vi "Teleop.vi"(10 "Match Info":T1={"Autonomous Elapsed Seconds"=0.0, "TeleOp Elapsed Seconds"=0.0, "Disabled Elapsed Seconds"=0.0, "Visited Autonomous"=FALSE, "Visited TeleOp"=FALSE, "Visited Disabled"=FALSE, "Autonomous Settings"={"Autonomous Style"=enum."Independent", "VI Refnum"=refnum}}, 11 "Call Context":T2) -> ()   [LabVIEW 2015]
doc: "This VI is called for each TeleOp packet received from the DS where the robot is not disabled. It is often used to read from the joysticks and update I/O or to update setpoints for timed control loops. It should complete and return within 20 milliseconds or it may miss DS packets."
uses:
  Robot Global Data.vi
  AppleScript/AppleScript Global Data.vi
  <vilib>/Rock Robotics/Network Tables/NT Read Number.vi
  <vilib>/Rock Robotics/WPI/DriverStation/WPI_DriverStationMatch Info.ctl
  <vilib>/Rock Robotics/WPI/DriverStation/WPI_DriverStationDerivedRobotMode.ctl
panel:
  out "Distance":dbl
  in  "reset":bool
  out "Yaw":dbl
  in  "milliseconds to wait":u32=10
  out "x-y":u32
  in  "inactive":dbl=1.0
  in  "active":dbl
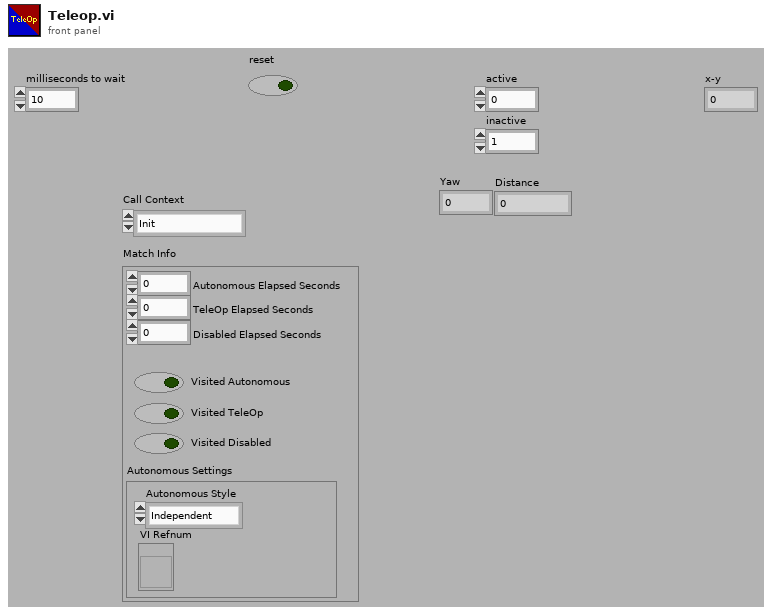
[diagram p1: front panel]
types:
  T1 = typedef "WPI_DriverStationMatch Info.ctl" = cluster{"Autonomous Elapsed Seconds":dbl, "TeleOp Elapsed Seconds":dbl, "Disabled Elapsed Seconds":dbl, "Visited Autonomous":bool, "Visited TeleOp":bool, "Visited Disabled":bool, "Autonomous Settings":cluster{"Autonomous Style":enum16{"Iterative", "Independent"}, "VI Refnum":refnum<vi>}}
  T2 = typedef "WPI_DriverStationDerivedRobotMode.ctl" = enum16{"Init", "Execute", "Stop"}
  T3 = typedef "WPI_JoystickDevRef.ctl" = cluster{"Device":T4}
  T4 = typedef "WPI_JoystickDeviceEnum.ctl" = enum16{"USB 0", "USB 1", "USB 2", "USB 3", "USB 4", "USB 5"}
  T5 = typedef "WPI_RobotDriveDevRef.ctl" = cluster{"DevStatus":errorcluster, "Motors[]":T6[], "Square Inputs":bool, "Max Output":dbl}
  T6 = typedef "WPI_MotorControlDeviceRef.ctl" = cluster{"DeviceStatus":errorcluster, "Type":T7, "PWM":cluster{"PWM Channel":T8, "DeadBand":T9}, "CAN":cluster{"Device Number":u8, "Control Mode":T10, "Semaphore":T11, "Max Vout":dbl, "TalonSRX Control Mode":T12}, "Invert":bool}
  T7 = typedef "WPI_MotorControlType.ctl" = enum16{"PWM", "CAN", "CANTalonSRX"}
  T8 = typedef "FPGA_DIOPWMChannel.ctl" = enum8{"PWM 0", "PWM 1", "PWM 2", "PWM 3", "PWM 4", "PWM 5", "PWM 6", "PWM 7", "PWM 8", "PWM 9", "PWM MXP 0", "PWM MXP 1", "PWM MXP 2", "PWM MXP 3", "PWM MXP 4", "PWM MXP 5", "PWM MXP 6", "PWM MXP 7", "PWM MXP 8", "PWM MXP 9", "Invalid"}
  T9 = typedef "WPI_PWMDeadband.ctl" = cluster{"Name":string, "maxPositivePwm":i32, "minPositivePwm":i32, "centerPwm":i32, "maxNegativePwm":i32, "minNegativePwm":i32, "angularRange":u16}
  T10 = typedef "WPI_CANJaguar_ControlMode.ctl" = enum8{"Percent VBus", "Current", "Speed", "Position", "Voltage"}
  T11 = typedef "Semaphore RefNum" = refnum<k1>
  T12 = typedef "WPI_CANTalonSRX_APIControlMode.ctl" = enum8{"Percent VBus", "Speed", "Position", "Slave", "Unchanged / Invalid", "Voltage Compensation", "Current", "Motion Profile"}
  T13 = typedef "WPI_ServoDeviceRef.ctl" = cluster{"DeviceStatus":errorcluster, "PWM Channel":T8, "DeadBand":T9}
  T14 = typedef "navX Library v2.lvlib/Z900_navX_DeviceTypeDef.ctl" = cluster{"Interface":cluster{"Protocol":T15, "Update Rate (4Hz-60Hz)":u8, "navX Open TypeDef":variant}, "Notify Packet":refnum<notifier>, "Loop VI Refnum":refnum<vi>, "Ready to Close Occurrence Refnum":refnum<k4>}
  T15 = typedef "navX Library v2.lvlib/Z900_navX_ProtocolTypeDef.ctl" = enum16{"SERIAL", "I2C", "SPI"}
  T16 = typedef "WPI_EncoderDevRef.ctl" = cluster{"DevStatus":errorcluster, "EncoderIndex":T17, "CounterIndex":T18, "DistancePerCount":dbl, "Decoding Type":T19}
  T17 = typedef "FPGA_EncoderIdx.ctl" = enum8{"Enc 0", "Enc 1", "Enc 2", "Enc 3", "Enc 4", "Enc 5", "Enc 6", "Enc 7", "Invalid"}
  T18 = typedef "FPGA_CounterCtrSystemIndex.ctl" = enum8{"Ctr 0", "Ctr 1", "Ctr 2", "Ctr 3", "Ctr 4", "Ctr 5", "Ctr 6", "Ctr 7", "Invalid"}
  T19 = typedef "WPI_EncoderType.ctl" = enum16{"1x", "2x", "4x"}
  T20 = cluster{"Yaw":dbl, "Roll":dbl, "Pitch":dbl, "Heading":dbl, "Fused Heading":dbl}
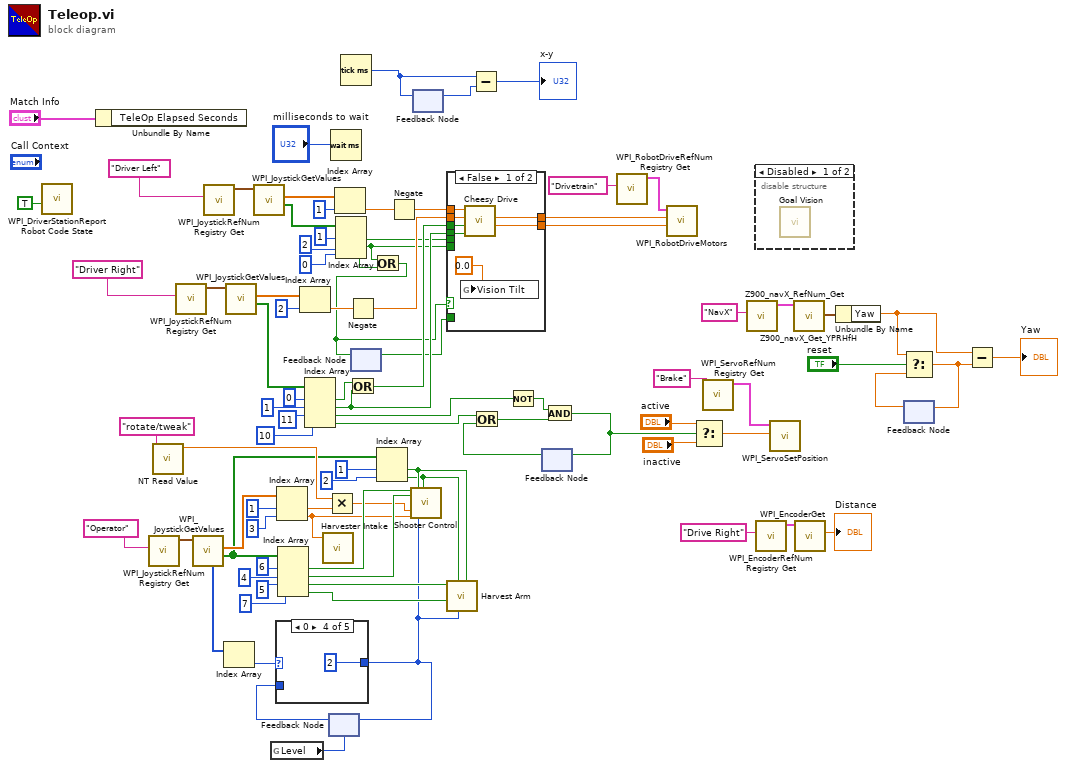
[diagram p0: block diagram]
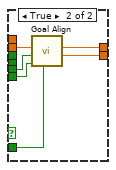
[diagram p3: hidden frame]
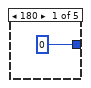
[diagram p4: hidden frame]
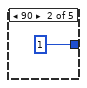
[diagram p5: hidden frame]
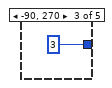
[diagram p6: hidden frame]
diagram:
  n1 = call <vilib>:"WPI_DriverStationReport Robot Code State.vi"("TeleOp"=TRUE ("Autonomous")) -> ()  [unwired: 10 in, 1 out]
  n2 = Unbundle By Name("Match Info") -> ()  [unwired: 1 out]
  n3 = call <vilib>:"WPI_JoystickRefNum Registry Get.vi"("refnum name"="Operator") -> ("JoystickDevRef"=w63:T3)  [unwired: 9 in, 1 out]
  n4 = call-poly <vilib>:"NT Read Value.vi"("Name"="rotate/tweak") -> ("Numeric"=w59:dbl)  [unwired: 9 in, 1 out]
  n5 = call <vilib>:"WPI_JoystickRefNum Registry Get.vi"("refnum name"="Driver Right") -> ("JoystickDevRef"=w83:T3)  [unwired: 1 in, 9 out]
  n6 = call <vilib>:"WPI_JoystickGetValues.vi"("JoystickDevRef"=w63) -> ("Buttons"=w52:bool[], "Axes"=w64:dbl[], "POVs"=w70:i16[])  [unwired: 6 in, 2 out]
  n7 = call <vilib>:"WPI_JoystickRefNum Registry Get.vi"("refnum name"="Driver Left") -> ("JoystickDevRef"=w87:T3)  [unwired: 1 in, 9 out]
  n8 = Index Array(array=w70) -> (element=w71:i16)  [unwired: 1 in]
  n9 = call <vilib>:"WPI_JoystickGetValues.vi"("JoystickDevRef"=w83) -> ("Buttons"=w30:bool[], "Axes"=w84:dbl[])  [unwired: 6 in, 3 out]
  n10 = call <vilib>:"WPI_JoystickGetValues.vi"("JoystickDevRef"=w87) -> ("Buttons"=w19:bool[], "Axes"=w85:dbl[])  [unwired: 6 in, 3 out]
  n11 = global read "AppleScript Global Data.vi" "Level"() -> (w8:i32)
  n12 = Index Array(array=w64, index #1=1 ("index"), index #2=3 ("index")) -> (element #1=w61:dbl, element #2=w54:dbl)
  n13 = Index Array(array=w52, index #1=6 ("index"), index #2=4 ("index"), index #3=5 ("index"), index #4=7 ("index")) -> (element #1=w69:bool, element #2=w73:bool, element #3=w56:bool, element #4=w55:bool)
  n14 = Index Array(array=w84, index=2) -> (element=w74:dbl)
  n15 = Index Array(array=w30, index #1=0 ("index"), index #2=1 ("index"), index #3=11 ("index"), index #4=10 ("index")) -> (element #1=w33:bool, element #2=w31:bool, element #3=w35:bool, element #4=w36:bool)
  n16 = call "Harvester Intake.vi"("Joy Val"=w54) -> ()  [unwired: 3 in]
  n17 = Multiply(x=w59, y=w61) -> (x*y=w27:dbl)
  n18 = feedback #1(w8) -> (w72:i32)
  n19 = case shown="0" w71 {
    tunnel: [0 ("index") 1 ("index") 3 ("index") 2 ("index") w94] -> w9
    tunnel: w72 -> [_ _ _ _ w94]
    frame 180 {
    }
    frame 90 {
    }
    frame -90, 270 {
    }
    frame 0 {
    }
    frame Default {
    }
  }
  n20 = feedback-in #1(w9) -> ()
  n21 = Wait (ms)(milliseconds to wait="milliseconds to wait") -> ()  [unwired: 1 out]
  n22 = Index Array(array=w85, index=1) -> (element=w20:dbl)
  n23 = Index Array(array=w19, index #1=1 ("index"), index #2=2 ("index"), index #3=0 ("index")) -> (element #1=w17:bool, element #2=w3:bool, element #3=w2:bool)
  n24 = Tick Count (ms)() -> (millisecond timer value=w39:u32)
  n25 = Negate(x=w74) -> (-x=w51:dbl)
  n26 = Or(x=w33, y=w31) -> (x .or. y?=w32:bool)
  n27 = feedback #2() -> (w24:bool)  [unwired: 1 in]
  n28 = Or(x=w3, y=w2) -> (x .or. y?=w1:bool)
  n29 = feedback-in #2(w1) -> ()
  n30 = Index Array(array=w52, index #1=1 ("index"), index #2=2 ("index")) -> (element #1=w29:bool, element #2=w28:bool)
  n31 = Negate(x=w20) -> (-x=w7:dbl)
  n32 = call "Shooter Control.vi"("Shooter Wheel On?"=w69, "Fire"=w73, "Rotate Tweak"=w27, "Harvester Axis"=w54, "duck"=w29, "Shooter Arm Level"=w9, "low goal"=w28) -> ()  [unwired: 13 in]
  n33 = feedback-in #3(w39) -> ()
  n34 = feedback #3() -> (w40:u32)  [unwired: 1 in]
  n35 = case shown="False" w1 {
    tunnel: [w101 w107] -> w76
    tunnel: [w100 w106] -> w75
    tunnel: w7 -> [w99 _]
    tunnel: w51 -> [w98 w102]
    tunnel: w32 -> [w97 _]
    tunnel: w31 -> [w96 _]
    tunnel: w24 -> [_ w105]
    tunnel: w17 -> [_ w104]
    tunnel: w3 -> [_ w103]
    frame False {
      n36 = global write "Robot Global Data.vi" "Vision Tilt"(0.0) -> ()
      n37 = call "Cheesy Drive.vi"("Slow turn"=w96, "Quickturn"=w97, "Turn"=w98, "Throttle"=w99) -> ("Right"=w100:dbl, "Left"=w101:dbl)  [unwired: 4 in]
    }
    frame True {
      n38 = call "Goal Align.vi"("Turn offset"=w102, "override shooter"=w104, "override drive"=w103, "last"=w105) -> ("Left"=w107:dbl, "Right"=w106:dbl)  [unwired: 4 in, 1 out]
    }
  }
  n39 = call "Harvest Arm.vi"("Lift Mode"=w29, "Level"=w9, "Low Goal"=w28, "Arm Down"=w55, "Arm Up"=w56) -> ()  [unwired: 7 in]
  n40 = Subtract(x=w39, y=w40) -> (x-y=→"x-y":u32)
  n41 = Not(x=w35) -> (.not. x?=w46:bool)
  n42 = feedback #4() -> (w45:bool)  [unwired: 1 in]
  n43 = Or(x=w36, y=w45) -> (x .or. y?=w47:bool)
  n44 = And(x=w46, y=w47) -> (x .and. y?=w44:bool)
  n45 = feedback-in #4(w44) -> ()
  n46 = call <vilib>:"WPI_RobotDriveRefNum Registry Get.vi"("refnum name"="Drivetrain") -> ("RobotDriveDevRef"=w78:T5)  [unwired: 9 in, 1 out]
  n47 = call <vilib>:"WPI_RobotDriveMotors.vi"("RightSpeed"=w75, "LeftSpeed"=w76, "RobotDriveDevRef"=w78) -> ()  [unwired: 6 in, 3 out]
  n48 = Select(t="active", s=w44, f="inactive") -> (s? t:f=w25:dbl)
  n49 = call <vilib>:"WPI_ServoRefNum Registry Get.vi"("refnum name"="Brake") -> ("ServoDeviceRef"=w26:T13)  [unwired: 9 in, 1 out]
  n50 = call "Z900_navX_RefNum_Get.vi"("refnum name"="NavX") -> ("navX Device"=w21:T14)  [unwired: 9 in, 1 out]
  n51 = disable-structure shown="Disabled" {
    frame Disabled {
      n52 = call "Goal Vision.vi"() -> ()  [unwired: 8 in, 3 out]
    }
    frame Enabled {
    }
  }
  n53 = call <vilib>:"WPI_EncoderRefNum Registry Get.vi"("refnum name"="Drive Right") -> ("EncoderDevRef"=w6:T16)  [unwired: 9 in, 1 out]
  n54 = call <vilib>:"WPI_ServoSetPosition.vi"("Position"=w25, "ServoDeviceRef"=w26) -> ()  [unwired: 8 in, 2 out]
  n55 = call "Z900_navX_Get_YPRHfH.vi"("navX Device"=w21) -> ("YRPHfH"=w22:T20)  [unwired: 7 in, 3 out]
  n56 = call <vilib>:"WPI_EncoderGet.vi"("EncoderDevRef"=w6) -> ("Distance"=→"Distance":dbl)  [unwired: 5 in, 5 out]
  n57 = Unbundle By Name(w22) -> ("Yaw"=w11:dbl)
  n58 = feedback #5() -> (w13:dbl)  [unwired: 1 in]
  n59 = Select(t=w11, s="reset", f=w13) -> (s? t:f=w10:dbl)
  n60 = feedback-in #5(w10) -> ()
  n61 = Subtract(x=w11, y=w10) -> (x-y=→"Yaw":dbl)
